vi "ABR3-Adapt Number of Averages.vi"(0 "Runtime":T1={"Ceiling"=0.0, "Threshold"=0.0, "Crossed?"=FALSE, "Step"=0, "Stop"=0, "Avgs"=0, "Level"=0.0, "AI Npts"=0, "Doubled?"=FALSE, "Gain"=0.0, "NWindowPts"=0, "dt"=0.0, "Cal"=path "", "Freq"=0.0, "AO Channels"=[], "AltPol"=FALSE, "AO Npts"=0, "AO Fs"=0.0, "Start"=0, "Stop max"=0, "Ear"=enum."Right", "Waveform"=enum."TONE PIP", "RepRate"=0.0, "CAP or ABR"=1, "LMasker"=0.0, "SeqVar"=enum."Signal Level", "Reps/buffer"=0, "Avg Mode"=enum."Neural/CM", "Wav"=path "", "Order"=enum."Sequential", "Levels"=[], "ControlVal"=0.0, "innerIndex"=0, "indexStep"=0} {"CAP or ABR" items=["CAP", "ABR"]}, 5 "Amplitude":dbl, 11 "error in (no error)":errorcluster) -> (4 "Runtime out":T1={"Ceiling"=0.0, "Threshold"=0.0, "Crossed?"=FALSE, "Step"=0, "Stop"=0, "Avgs"=0, "Level"=0.0, "AI Npts"=0, "Doubled?"=FALSE, "Gain"=0.0, "NWindowPts"=0, "dt"=0.0, "Cal"=path "", "Freq"=0.0, "AO Channels"=[], "AltPol"=FALSE, "AO Npts"=0, "AO Fs"=0.0, "Start"=0, "Stop max"=0, "Ear"=enum."Right", "Waveform"=enum."TONE PIP", "RepRate"=0.0, "CAP or ABR"=1, "LMasker"=0.0, "SeqVar"=enum."Signal Level", "Reps/buffer"=0, "Avg Mode"=enum."Neural/CM", "Wav"=path "", "Order"=enum."Sequential", "Levels"=[], "ControlVal"=0.0, "innerIndex"=0, "indexStep"=0} {"CAP or ABR" items=["CAP", "ABR"]}, 15 "error out":errorcluster)   [LabVIEW 2020]
uses:
  TypeDefs/ABR3-Runtime Data.ctl
  epl-vi-lib/Utility VIs/Type Defs/Left-Right ring.ctl
  TypeDefs/ABR-Waveform Enum.ctl
  TypeDefs/ABR3-Seq Var Enum.ctl
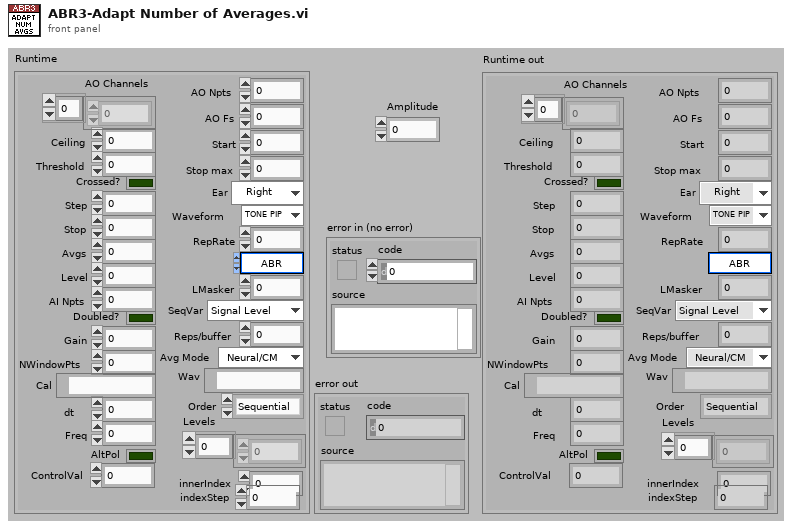
[diagram p1: front panel]
types:
  T1 = typedef "ABR3-Runtime Data.ctl" = cluster{"Ceiling":dbl, "Threshold":dbl, "Crossed?":bool, "Step":i32, "Stop":i32, "Avgs":i32, "Level":dbl, "AI Npts":i32, "Doubled?":bool, "Gain":dbl, "NWindowPts":i32, "dt":dbl, "Cal":path, "Freq":dbl, "AO Channels":i32[], "AltPol":bool, "AO Npts":i32, "AO Fs":dbl, "Start":i32, "Stop max":i32, "Ear":T2, "Waveform":T3, "RepRate":dbl, "CAP or ABR":u16, "LMasker":dbl, "SeqVar":T4, "Reps/buffer":i32, "Avg Mode":enum16{"Neural/CM", "ANOW"}, "Wav":path, "Order":enum16{"Sequential", "Random"}, "Levels":dbl[], "ControlVal":dbl, "innerIndex":i32, "indexStep":i32}
  T2 = typedef "Left-Right ring.ctl" = enum16{"Right", "Left"}
  T3 = typedef "ABR-Waveform Enum.ctl" = enum16{"TONE PIP", "CLICK", "FILE", "CHIRP", "NOISE", "VERHULST"}
  T4 = typedef "ABR3-Seq Var Enum.ctl" = enum16{"Signal Level", "Masker Level"}
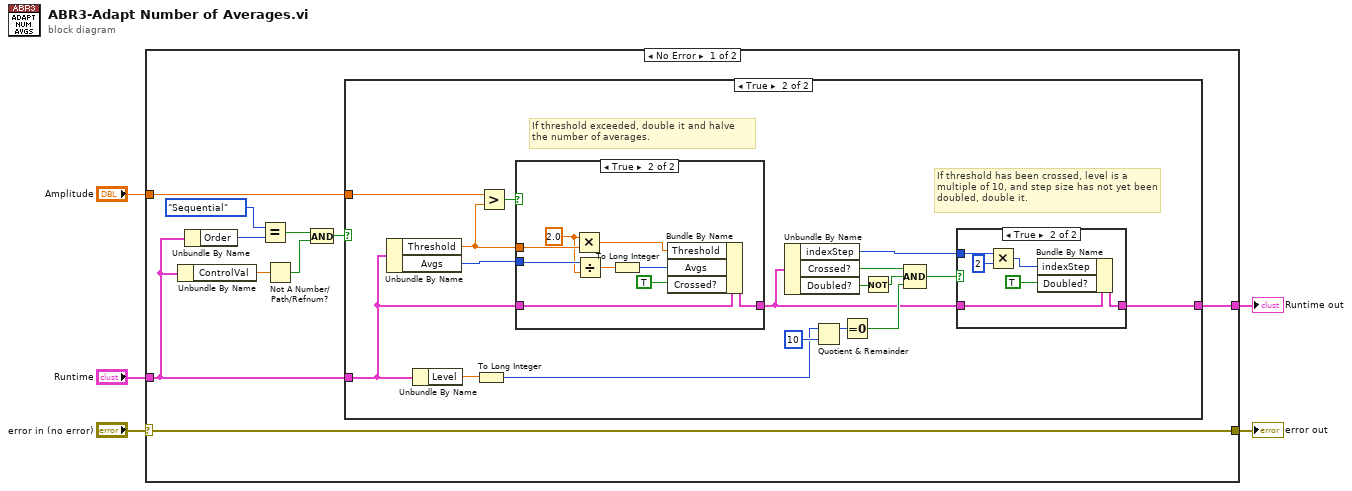
[diagram p0: block diagram]
diagram:
  n1 = case shown="No Error" "error in (no error)" {
    selector: "error in (no error)" -> [w14 w51]
    tunnel: "Runtime" -> [w9 w52]
    tunnel: "Amplitude" -> [w15 _]
    tunnel: [w13 w52] -> w2
    tunnel: [w14 w51] -> w1
    frame No Error {
      n2 = Unbundle By Name(w9) -> ("ControlVal"=w8:dbl)
      n3 = Unbundle By Name(w9) -> ("Order"=w11:enum16{"Sequential", "Random"})
      n4 = Equal?(x=enum16{"Sequential", "Random"}."Sequential" ("y"), y=w11) -> (x = y?=w12:bool)
      n5 = Not A Number/Path/Refnum?(number/path/refnum=w8) -> (NaN/Path/Refnum?=w6:bool)
      n6 = And(x=w12, y=w6) -> (x .and. y?=w7:bool)
      n7 = case shown="True" w7 {
        tunnel: w15 -> [_ w33]
        tunnel: w9 -> [w16 w28]
        tunnel: [w16 w17] -> w13
        frame False {
        }
        frame True {
          # "If threshold has been crossed, level is a multiple of 10, and step size has not yet been doubled, double it."
          # "If threshold exceeded, double it and halve the number of averages."
          n8 = Unbundle By Name(w28) -> ("Threshold"=w30:dbl, "Avgs"=w29:i32)
          n9 = Unbundle By Name(w28) -> ("Level"=w27:dbl)
          n10 = To Long Integer(number=w27) -> (32bit integer=w25:i32)
          n11 = Greater?(x=w33, y=w30) -> (0:w26:bool)
          n12 = case shown="True" w26 {
            tunnel: w28 -> [w41 w43]
            tunnel: w30 -> [_ w50]
            tunnel: w29 -> [_ w49]
            tunnel: [w41 w45] -> w18
            frame False {
            }
            frame True {
              w48 = 2.0 ("y")
              n13 = Multiply(x=w48, y=w50) -> (x*y=w47:dbl)
              n14 = Divide(x=w49, y=w48) -> (x/y=w46:dbl)
              n15 = To Long Integer(number=w46) -> (32bit integer=w44:i32)
              n16 = Bundle By Name(cluster=w43, "Threshold"=w47, "Avgs"=w44, "Crossed?"=TRUE) -> (w45:T1)
            }
          }
          n17 = Unbundle By Name(w18) -> ("indexStep"=w19:i32, "Crossed?"=w23:bool, "Doubled?"=w24:bool)
          n18 = Quotient & Remainder(x=w25, y=10) -> (x-y*floor(x/y)=w31:i32)  [unwired: 1 out]
          n19 = Equal To 0?(x=w31) -> (x = 0?=w21:bool)
          n20 = Not(x=w24) -> (.not. x?=w22:bool)
          n21 = Compound Arithmetic op=AND(w23, w22, w21) -> (w20:bool)
          n22 = case shown="True" w20 {
            tunnel: [w34 w37] -> w17
            tunnel: w19 -> [_ w36]
            tunnel: w18 -> [w34 w35]
            frame False {
            }
            frame True {
              n23 = Multiply(x=w36, y=2) -> (x*y=w39:i32)
              n24 = Bundle By Name(cluster=w35, "indexStep"=w39, "Doubled?"=TRUE ("Crossed?")) -> (w37:T1)
            }
          }
        }
      }
    }
    frame Error {
    }
  }
  "error out" <- w1
  "Runtime out" <- w2
